vi "View.vi"(8 "error in (no error)":errorcluster, 10 "Debugger":refnum<class "Debug Process.lvclass">, 11 "List View In":refnum<class "Processes List Box View.lvclass">) -> (0 "error out":errorcluster)   [LabVIEW 2020, in "Processes List Box View.lvclass"]
uses:
  Processes List Box View.lvclass
  C:/Users/anton/Documents/GitHub/triarc-debugger/source/Debug View/Debug View.lvclass
  Process/Debug Process.lvclass
  Debug View/Debug View.lvclass/Debug View.ctl
  Processes List Box View.lvclass/Processes List Box View.ctl
  Debugger/Debugger.lvclass
  List Box View Model_/List Box View Model.lvclass
  Debug View/Debug View.lvclass
panel:
  in  "Listbox":i32[](listbox)
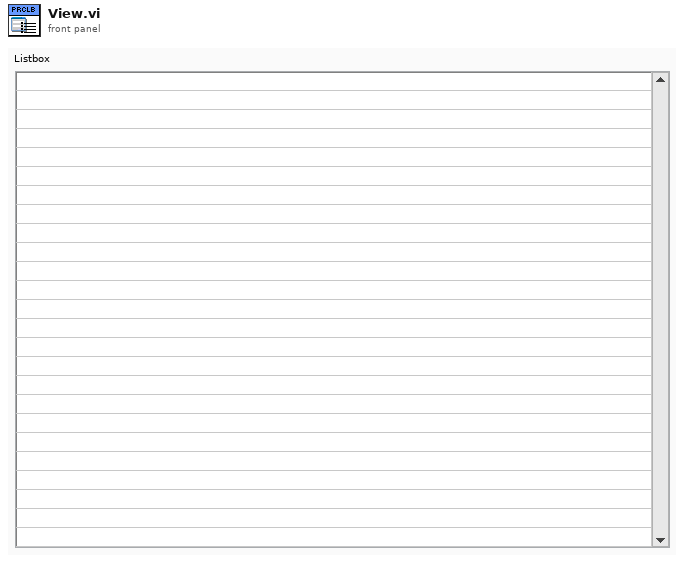
[diagram p1: front panel]
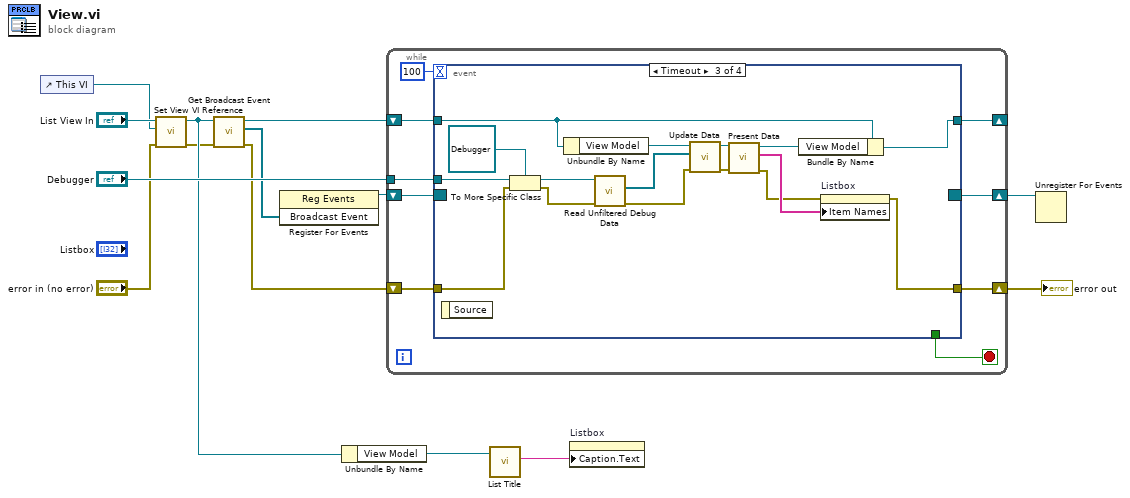
[diagram p0: block diagram]
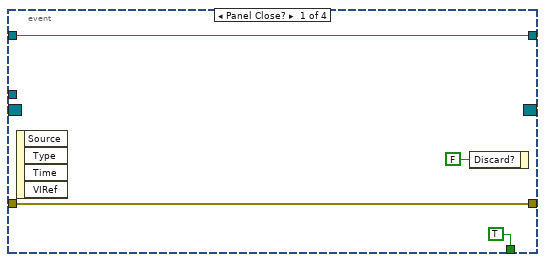
[diagram p2: hidden frame]
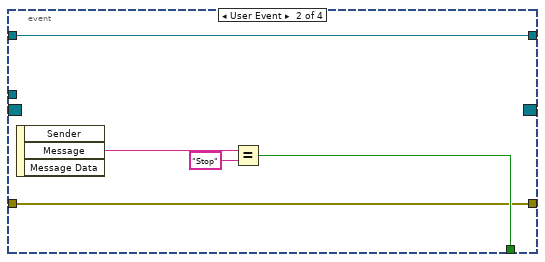
[diagram p3: hidden frame]
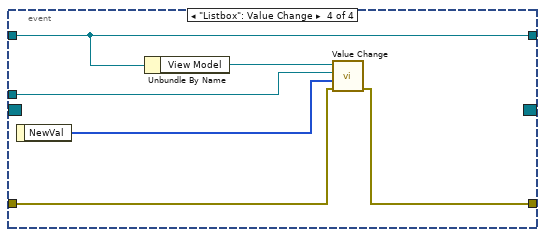
[diagram p4: hidden frame]
diagram:
  n1 = control-ref of="This VI"() -> (w4:refnum<vi>)
  n2 = call "Set View VI Reference.vi"("error in (no error)"="error in (no error)", "View VI ref"=w4, "Debug View in"="List View In") -> ("error out"=w2:errorcluster, "Debug View out"=w5:refnum<class "Processes List Box View.lvclass">)  [unwired: 7 in]
  n3 = call "Get Broadcast Event.vi"("error in (no error)"=w2, "Debug View In"=w5) -> ("error out"=w1:errorcluster, "Broadcast Event"=w6:refnum<user-event>[], "Debug View Out"=w7:refnum<class "Processes List Box View.lvclass">)  [unwired: 7 in]
  n4 = register-events(w6) -> (reference out=w9:refnum<event-registration>)  [unwired: 2 in, 1 out]
  n5 = Unbundle By Name(w5) -> ("View Model"=w12:refnum<class "List Box View Model.lvclass">)
  n6 = while {
    shift-right: [w22] -> _
    shift-left: w7 -> [w23]
    shift-right: [w21] -> w14
    shift-left: w1 -> [w20]
    shift-right: [w19] -> w13
    shift-left: w9 -> [w18]
    tunnel: "Debugger" -> [w17]
    stop <- w16 stop-if-true
    n7 = event shown="[2] Timeout" {
      selector: w18 -> [_ _ _ _]
      dyn-events: [_ _ _ _] -> w19
      timeout: 100 -> [_ _ _ _]
      tunnel: w23 -> [w27 w28 w41 w54]
      tunnel: [w27 w28 w40 w54] -> w22
      tunnel: [w26 w29 w33 w50] -> w21
      tunnel: w20 -> [w26 w29 w44 w49]
      tunnel: w17 -> [_ _ w42 w52]
      tunnel: [TRUE ("Discard?") w30 _ _] -> w16
      event Panel Close? {
        n8 = event-data() -> ()  [unwired: 1 in, 4 out]
        n9 = event-data("Discard?"=FALSE) -> ()  [unwired: 1 in, 1 out]
      }
      event User Event {
        n10 = event-data() -> ("Message"=w32:string)  [unwired: 1 in, 2 out]
        n11 = Equal?(x=w32, y="Stop") -> (x = y?=w30:bool)
      }
      event Timeout {
        n12 = event-data() -> ()  [unwired: 1 in, 1 out]
        n13 = To More Specific Class(target class=refnum<class "Debugger.lvclass"> refnum ("Debugger.lvclass"), reference=w42, error in=w44) -> (specific class reference=w39:refnum<class "Debugger.lvclass">, error out=w38:errorcluster)
        n14 = Unbundle By Name(w41) -> ("View Model"=w48:refnum<class "List Box View Model.lvclass">)
        n15 = call "Read Unfiltered Debug Data.vi"("error in (no error)"=w38, "Debugger In"=w39) -> ("error out"=w36:errorcluster, "Data Log"=w37:refnum<class "Debug Data.lvclass">[])  [unwired: 7 in, 1 out]
        n16 = call-dynamic "Update Data.vi"("error in (no error)"=w36, "Debug Data"=w37, "List Seen Processes View Model In"=w48) -> ("error out"=w35:errorcluster, "List Seen Processes View Model Out"=w45:refnum<class "List Box View Model.lvclass">)  [unwired: 7 in]
        n17 = call "Present Data.vi"("error in (no error)"=w35, "List Seen Processes View Model In"=w45) -> ("error out"=w34:errorcluster, "Message List"=w47:string[], "List Seen Processes View Model Out"=w46:refnum<class "List Box View Model.lvclass">)  [unwired: 7 in]
        n18 = Bundle By Name(cluster=w41, "View Model"=w46) -> (w40:refnum<class "Processes List Box View.lvclass">)
        n19 = property on="Listbox" class="LstBox (strict)"(error in=w34, "Item Names"=w47) -> (error out=w33:errorcluster)  [unwired: 1 in, 1 out]
      }
      event "Listbox": Value Change {
        n20 = event-data() -> ("NewVal"=w51:i32[])  [unwired: 1 in]
        n21 = Unbundle By Name(w54) -> ("View Model"=w53:refnum<class "List Box View Model.lvclass">)
        n22 = call-dynamic "Value Change.vi"("error in (no error)"=w49, "NewVal"=w51, "Debugger"=w52, "List Box View Model In"=w53) -> ("error out"=w50:errorcluster)  [unwired: 6 in, 1 out]
      }
    }
  }
  "error out" <- w14
  n23 = call-dynamic "List Title.vi"("List Box View Model in"=w12) -> ("Title"=w11:string)  [unwired: 8 in, 2 out]
  n24 = property on="Listbox" class="LstBox (strict)"("Caption.Text"=w11) -> ()  [unwired: 2 in, 2 out]
  n25 = Unregister For Events(event registration refnum=w13) -> ()  [unwired: 1 in, 1 out]
